vi "format_python_cmd.vi"(11 "python cmd":string) -> (3 "system exec python cmd":string)   [LabVIEW 2018]
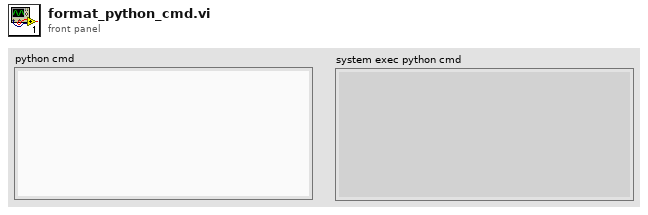
[diagram p1: front panel]
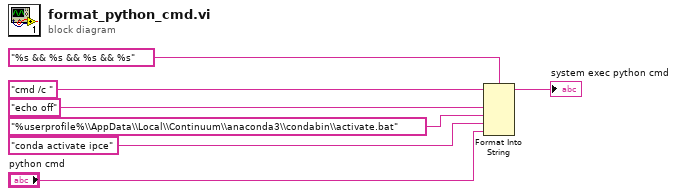
[diagram p0: block diagram]
diagram:
  n1 = Format Into String(format string="%s && %s && %s && %s", initial string="cmd /c ", "echo off" ("input 1"), "%userprofile%\\AppData\\Local\\Continuum\\anaconda3\\condabin\\activate.bat" ("input 2"), "conda activate ipce" ("input 2"), "python cmd") -> (resulting string=→"system exec python cmd":string)  [unwired: 1 in, 1 out]
